vi "simx Read Proximity Sensor.vi"(0 "clientID":i32, 1 "detectedObjectHandle":i32, 2 "operationMode":i32, 5 "sensorHandle":i32, 7 "detectionState":string, 9 "detectedPoint":sgl, 11 "error in (no error)":errorcluster, 12 "detectedSurfaceNormalVector":sgl) -> (3 "detectedObjectHandle out":i32, 4 "function return":i32, 8 "detectionState out":string, 10 "detectedPoint out":sgl, 14 "detectedSurfaceNormalVector out":sgl, 15 "error out":errorcluster)   [LabVIEW 2019, in "PXL_V-REP.lvlib"]
doc: "EXTAPI_DLLEXPORT simxInt simxReadProximitySensor(simxInt clientID,simxInt sensorHandle,simxUChar* detectionState,simxFloat* detectedPoint,simxInt* detectedObjectHandle,simxFloat* detectedSurfaceNormalVector,simxInt operationMode);"
uses:
  PXL_V-REP.lvlib
  <userlib>/V-REP/remoteApi.dll
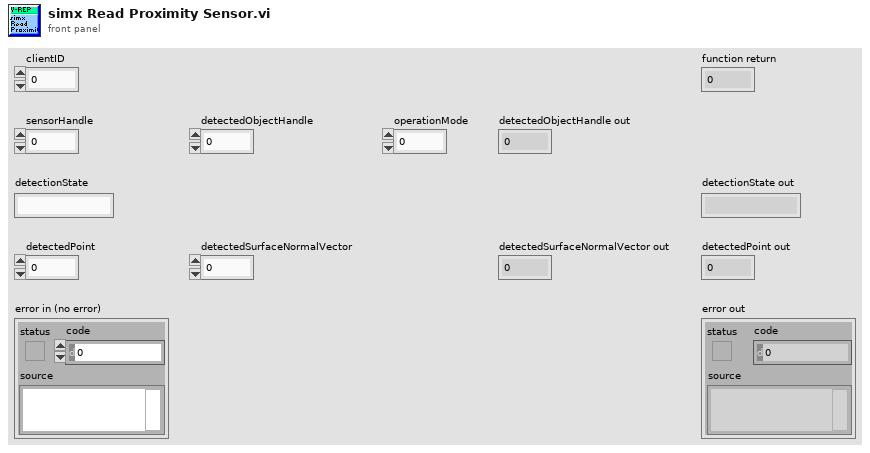
[diagram p1: front panel]
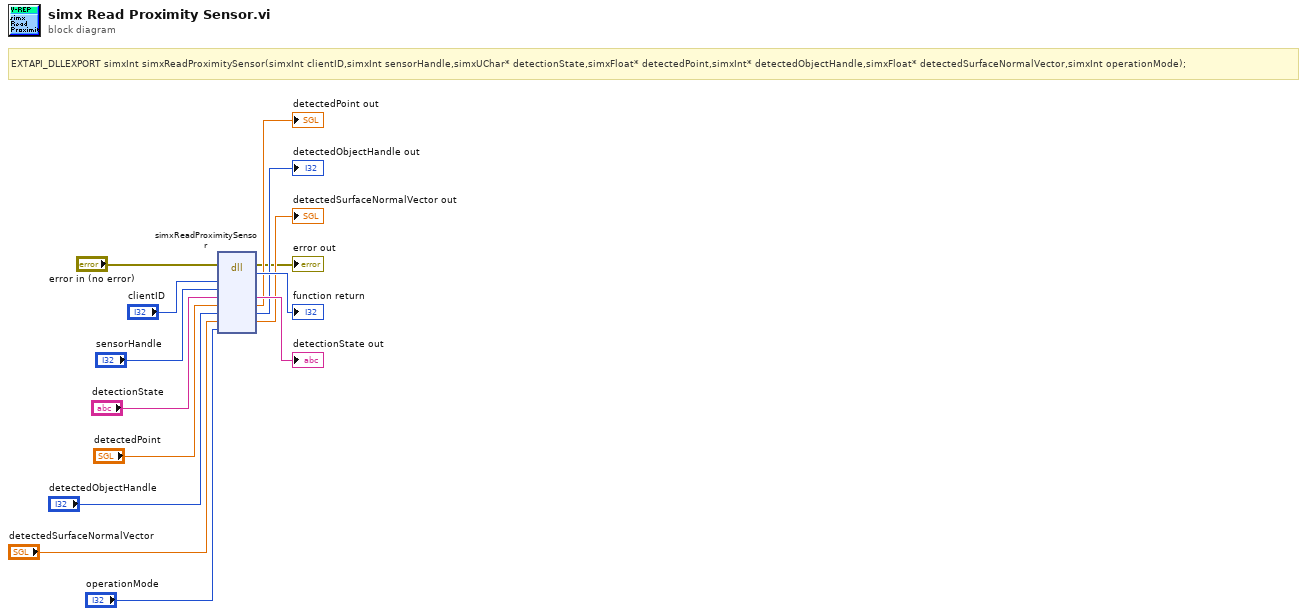
[diagram p0: block diagram]
diagram:
  # "EXTAPI_DLLEXPORT simxInt simxReadProximitySensor(simxInt clientID,simxInt sensorHandle,simxUChar* detectionState,simxFloat* detectedPoint,simxInt* detectedObjectHandle,simxFloat* detectedSurfaceNormalVector,simxInt operationMode);"
  n1 = dll-call lib="C:/Program Files (x86)/National Instruments/LabVIEW 2019/user.lib/V-REP/remoteApi.*" fn="simxReadProximitySensor"(error in="error in (no error)", "clientID"="clientID", "sensorHandle"="sensorHandle", "detectionState"="detectionState", "detectedPoint"="detectedPoint", "detectedObjectHandle"="detectedObjectHandle", "detectedSurfaceNormalVector"="detectedSurfaceNormalVector", "operationMode"="operationMode") -> (error out=→"error out":errorcluster, →"function return":i32, "detectionState"=→"detectionState out":string, "detectedPoint"=→"detectedPoint out":sgl, "detectedObjectHandle"=→"detectedObjectHandle out":i32, "detectedSurfaceNormalVector"=→"detectedSurfaceNormalVector out":sgl)  [unwired: 5 in, 1 out]
